vi "startSweepAndWait.vi"(8 "error in (no error)":errorcluster, 10 "setSweepConfiguration":variant, 11 "Instrument.LockinAPI in":refnum<class "Instrument.LockinAPI.lvclass">) -> (0 "error out":errorcluster, 1 "Results":T1, 2 "Waveforms":T2, 3 "Instrument.LockinAPI out":refnum<class "Instrument.LockinAPI.lvclass">)   [LabVIEW 2019, in "Instrument.LockinAPI.lvclass"]
uses:
  Instrument.LockinAPI.lvclass
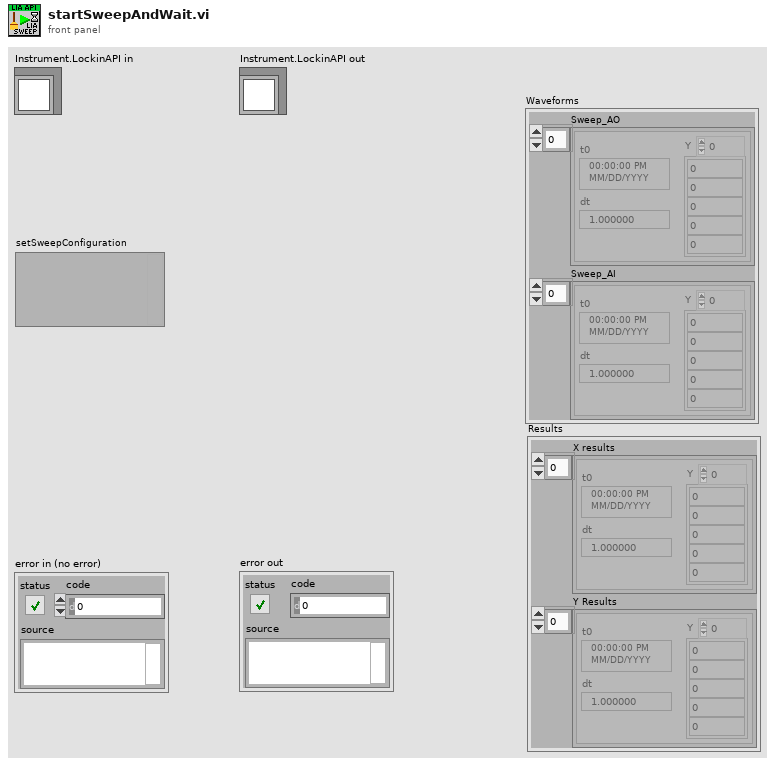
[diagram p1: front panel]
types:
  T1 = cluster{"X results":waveform(dbl)[], "Y Results":waveform(dbl)[]}
  T2 = cluster{"Sweep_AO":waveform(dbl)[], "Sweep_AI":waveform(dbl)[]}
  T3 = cluster{"Sweep Time (s)":dbl, "Initial Wait (s)":dbl, "Return to Start":bool, "Channels":cluster{"Enable?":bool, "Channel":u16, "Start":dbl, "End":dbl, "Pattern":enum16{"Ramp /", "Ramp /\\", "Smooth Ramp _/", "Smooth Ramp _/\\_", "Table"}, "Table":dbl[]}[]}
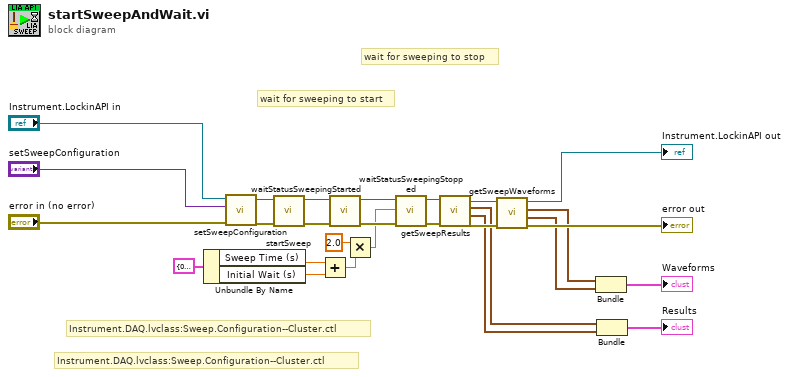
[diagram p0: block diagram]
diagram:
  # "Instrument.DAQ.lvclass:Sweep.Configuration--Cluster.ctl"
  # "Instrument.DAQ.lvclass:Sweep.Configuration--Cluster.ctl"
  # "wait for sweeping to stop"
  # "wait for sweeping to start"
  n1 = Unbundle By Name(T3 {"Sweep Time (s)"=0.0, "Initial Wait (s)"=0.0, "Return to Start"=FALSE, "Channels"=[]} ("input cluster")) -> ("Sweep Time (s)"=w12:dbl, "Initial Wait (s)"=w11:dbl)
  n2 = call-dynamic "setSweepConfiguration.vi"("error in (no error)"="error in (no error)", "setSweepConfiguration"="setSweepConfiguration", "Instrument.LockinAPI in"="Instrument.LockinAPI in") -> ("error out"=w25:errorcluster, "Instrument.LockinAPI out"=w26:refnum<class "Instrument.LockinAPI.lvclass">)  [unwired: 7 in]
  n3 = call "startSweep.vi"("error in (no error)"=w25, "Instrument.LockinAPI in"=w26) -> ("error out"=w18:errorcluster, "Instrument.LockinAPI out"=w23:refnum<class "Instrument.LockinAPI.lvclass">)  [unwired: 8 in]
  n4 = Add(x=w12, y=w11) -> (x+y=w10:dbl)
  n5 = call "waitStatusSweepingStarted.vi"("error in (no error)"=w18, "Instrument.LockinAPI in"=w23) -> ("error out"=w19:errorcluster, "Instrument.LockinAPI out"=w22:refnum<class "Instrument.LockinAPI.lvclass">)  [unwired: 8 in]
  n6 = Multiply(x=2.0, y=w10) -> (x*y=w8:dbl)
  n7 = call "waitStatusSweepingStopped.vi"("error in (no error)"=w19, "time (s) [10 s]"=w8, "Instrument.LockinAPI in"=w22) -> ("error out"=w20:errorcluster, "Instrument.LockinAPI out"=w21:refnum<class "Instrument.LockinAPI.lvclass">)  [unwired: 7 in]
  n8 = call-dynamic "getSweepResults.vi"("error in (no error)"=w20, "Instrument.LockinAPI in"=w21) -> ("error out"=w16:errorcluster, "Y Results"=w4:waveform(dbl)[], "X results"=w5:waveform(dbl)[], "Instrument.LockinAPI out"=w17:refnum<class "Instrument.LockinAPI.lvclass">)  [unwired: 6 in]
  n9 = call-dynamic "getSweepWaveforms.vi"("error in (no error)"=w16, "Instrument.LockinAPI in"=w17) -> ("error out"=→"error out":errorcluster, "Sweep_AI"=w6:waveform(dbl)[], "Sweep_AO"=w7:waveform(dbl)[], "Instrument.LockinAPI out"=→"Instrument.LockinAPI out":refnum<class "Instrument.LockinAPI.lvclass">)  [unwired: 6 in]
  n10 = Bundle("Sweep_AO"=w7, "Sweep_AI"=w6) -> (→"Waveforms":T2)  [unwired: 1 in]
  n11 = Bundle("X results"=w5, "Y Results"=w4) -> (→"Results":T1)  [unwired: 1 in]
